vi "Function.vi"(8 "error in (no error)":errorcluster, 10 "Value":ext, 11 "Two Terminal in":refnum<class "Reciprocal_EXT.lvclass">) -> (0 "error out":errorcluster, 2 "Result":ext, 3 "Two Terminal out":refnum<class "Reciprocal_EXT.lvclass">)   [LabVIEW 2021, in "Reciprocal_EXT.lvclass"]
uses:
  Reciprocal_EXT.lvclass
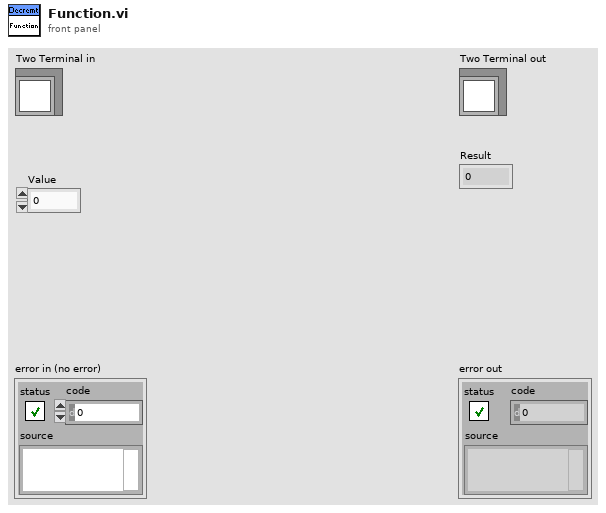
[diagram p1: front panel]
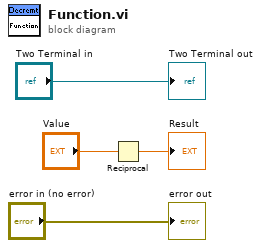
[diagram p0: block diagram]
diagram:
  n1 = Reciprocal(x="Value") -> (1/x=→"Result":ext)
  "error out" <- "error in (no error)"
  "Two Terminal out" <- "Two Terminal in"
